vi "Render to String.vi"(7 "Data":refnum<class "Abstract.lvclass">=refnum, 8 "Error In":errorcluster, 11 "Abstract Syntax Tree":refnum<class "Root.lvclass">=refnum) -> (0 "Error Out":errorcluster, 3 "Output":string)   [LabVIEW 2018, in "Toolkit.lvlib"]
uses:
  Toolkit.lvlib
  Data/Abstract/Abstract.lvclass
  Data/Map/Map.lvclass
  Data/String/String.lvclass
  Nodes/Root/Root.lvclass
  Nodes/Tag/Tag.lvclass
  Nodes/NonTerminal/NonTerminal.lvclass
  Nodes/Text/Text.lvclass
  Writers/String.lvclass
  D:/Users/cfield/Code/Field R&D Services/Mustache/trunk/src/Toolkit/Writers/Abstract/Abstract.lvclass
  Writers/String.lvclass/String.ctl
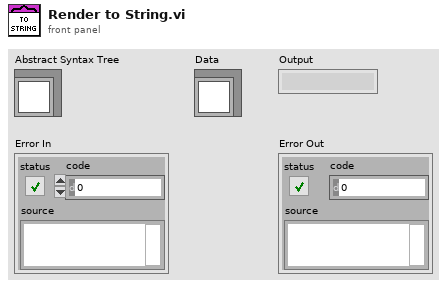
[diagram p1: front panel]
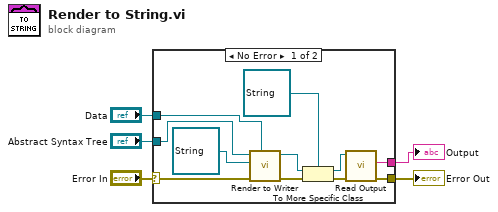
[diagram p0: block diagram]
diagram:
  n1 = case shown="No Error" "Error In" {
    selector: "Error In" -> [w15 w17]
    tunnel: [w14 w17] -> w4
    tunnel: [w13 _] -> w3
    tunnel: "Data" -> [w10 _]
    tunnel: "Abstract Syntax Tree" -> [w6 _]
    frame No Error {
      n2 = call "Render to Writer.vi"("Data"=w10, "Error In"=w15, "Writer In"=refnum<class "String.lvclass"> refnum ("Toolkit.lvlib:Writers.lvlib:String.lvclass"), "Abstract Syntax Tree"=w6) -> ("Error Out"=w16:errorcluster, "Writer Out"=w8:refnum<class "Abstract.lvclass">)  [unwired: 6 in]
      n3 = To More Specific Class(target class=refnum<class "String.lvclass"> refnum ("Toolkit.lvlib:Writers.lvlib:String.lvclass"), reference=w8, error in=w16) -> (specific class reference=w11:refnum<class "String.lvclass">, error out=w12:errorcluster)
      n4 = call "Read Output.vi"("Error In"=w12, "String In"=w11) -> ("Error Out"=w14:errorcluster, "Output"=w13:string)  [unwired: 7 in, 1 out]
    }
    frame Error {
    }
  }
  "Error Out" <- w4
  "Output" <- w3
